vi "SOFandEOF_del.vi"(8 "error in (no error)":errorcluster, 11 "Felica DOWN in":refnum<class "Felica DOWN.lvclass">) -> (0 "error out":errorcluster, 3 "Felica DOWN out":refnum<class "Felica DOWN.lvclass">)   [LabVIEW 2019, in "Felica DOWN.lvclass"]
uses:
  Felica DOWN.lvclass
  TypeDef/Store.ctl
  Felica DOWN.lvclass/Felica DOWN.ctl
  RFID system.lvclass
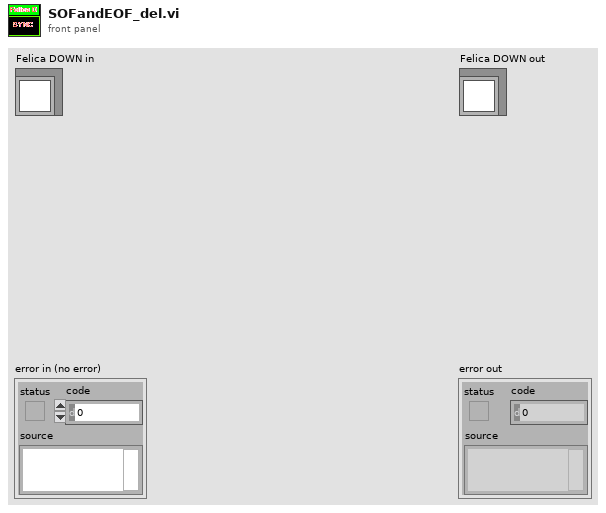
[diagram p1: front panel]
types:
  T1 = typedef "Store.ctl" = enum16{"envelope", "noise", "demSubCar", "CH_frame", "Decode", "demodulate", "in", "out", "sum", "subCarrier", "frame", "command", "encode", "modulate", "encode_UP", "modulate_up", "demod_up", "envelop_up", "sum_up", "out_up", "in_up"}
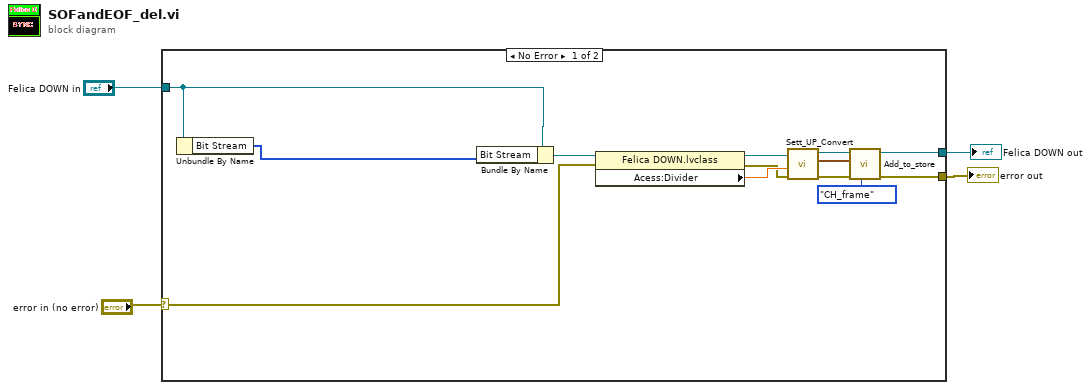
[diagram p0: block diagram]
diagram:
  n1 = case shown="No Error" "error in (no error)" {
    selector: "error in (no error)" -> [w7 w18]
    tunnel: "Felica DOWN in" -> [w17 w19]
    tunnel: [w14 w19] -> w2
    tunnel: [w12 w18] -> w1
    frame No Error {
      n2 = Unbundle By Name(w17) -> ("Bit Stream"=w5:u8[])
      n3 = Bundle By Name(cluster=w17, "Bit Stream"=w5) -> (w16:refnum<class "Felica DOWN.lvclass">)
      n4 = property class="Felica DOWN.lvclass"(reference=w16, error in=w7) -> (reference out=w9:refnum<class "Felica DOWN.lvclass">, error out=w6:errorcluster, "Acess:Divider"=w8:dbl)
      n5 = call-dynamic "Sett_UP_Convert.vi"("error in (no error)"=w6, "Divider(1)"=w8, "Felica DOWN in"=w9) -> ("error out"=w13:errorcluster, "Waveform"=w10:waveform(dbl), "Felica DOWN out"=w15:refnum<class "Felica DOWN.lvclass">)  [unwired: 6 in]
      n6 = call "Add_to_store.vi"("Store"=Store."CH_frame", "error in (no error)"=w13, "Waveform"=w10, "RFID system in"=w15) -> ("error out"=w12:errorcluster, "RFID system out"=w14:refnum<class "Felica DOWN.lvclass">)  [unwired: 6 in]
    }
    frame Error {
    }
  }
  "error out" <- w1
  "Felica DOWN out" <- w2
